vi "Set Backlash Compensation Motor.vi"(6 "Backlash Compensation Value (0 units)":dbl format="%.4g", 8 "error in (no error)":errorcluster, 9 "Axis (1)":i32=1 min=1 max=3, 10 "VISA resource name":refnum<visa-resource-name>, 11 "ESP301 in":refnum<class "ESP301.lvclass">) -> (0 "error out":errorcluster, 2 "VISA resource name out":refnum<visa-resource-name>, 3 "ESP301 out":refnum<class "ESP301.lvclass">)   [LabVIEW 2020, in "ESP301.lvclass"]
uses:
  ESP301.lvclass
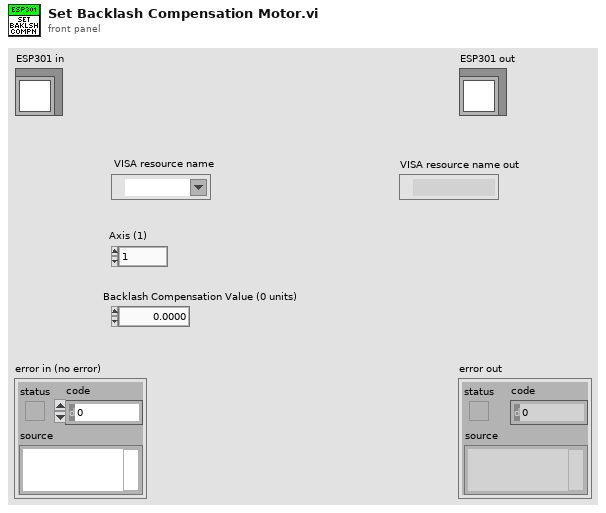
[diagram p1: front panel]
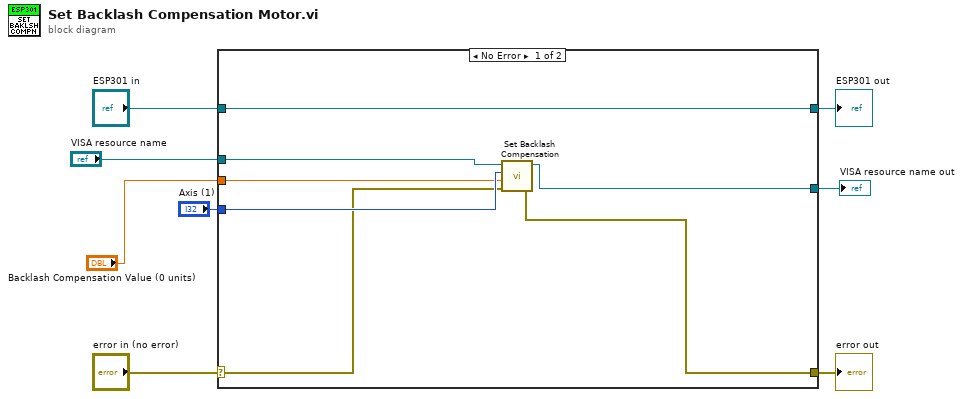
[diagram p0: block diagram]
diagram:
  n1 = case shown="No Error" "error in (no error)" {
    selector: "error in (no error)" -> [w10 w18]
    tunnel: [w9 w18] -> w7
    tunnel: [w15 w17] -> w5
    tunnel: "ESP301 in" -> [w15 w17]
    tunnel: "VISA resource name" -> [w14 w16]
    tunnel: [w13 w16] -> w3
    tunnel: "Axis (1)" -> [w12 _]
    tunnel: "Backlash Compensation Value (0 units)" -> [w11 _]
    frame No Error {
      n2 = call "Set Backlash Compensation.vi"("error in (no error)"=w10, "Backlash Compensation Value (0 units)"=w11, "Axis (1)"=w12, "VISA resource name"=w14) -> ("error out"=w9:errorcluster, "VISA resource name out"=w13:refnum<visa-resource-name>)  [unwired: 2 in]
    }
    frame Error {
    }
  }
  "error out" <- w7
  "ESP301 out" <- w5
  "VISA resource name out" <- w3
